vi "Get NMEA.vi"(8 "error in (no error)":errorcluster, 11 "VISA GPS in":refnum<class "VISA GPS.lvclass">) -> (0 "error out":errorcluster, 2 "NMEA":refnum<class "nmea.lvclass">, 3 "VISA GPS out":refnum<class "VISA GPS.lvclass">)   [LabVIEW 2020, in "nmea.lvlib" / "VISA GPS.lvclass"]
uses:
  VISA GPS.lvclass
  nmea/nmea.lvclass
  VISA GPS.lvclass/VISA GPS.ctl
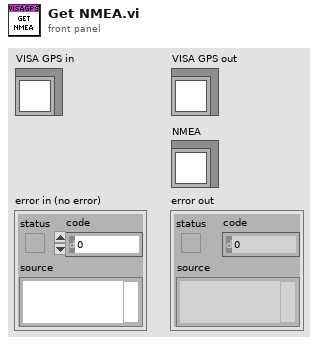
[diagram p1: front panel]
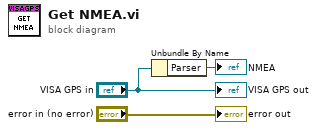
[diagram p0: block diagram]
diagram:
  n1 = Unbundle By Name("VISA GPS in") -> ("Parser"=→"NMEA":refnum<class "nmea.lvclass">)
  "error out" <- "error in (no error)"
  "VISA GPS out" <- "VISA GPS in"
